vi "Data Read old.vi"(8 "error in (no error)":errorcluster, 10 "Bytes To Read (256)":i32=256, 11 "VISA Refnum in":refnum<visa-resource-name>) -> (0 "error out":errorcluster, 2 "Response Cluster":T1 {"Command ID" format="%x"}, 3 "VISA Refnum out":refnum<visa-resource-name>, 5 "Response String (debug)":string)   [LabVIEW 2020, in "Omega Platinum Series.lvlib"]
uses:
  Omega Platinum Series.lvlib
  Type Defs/Response.ctl
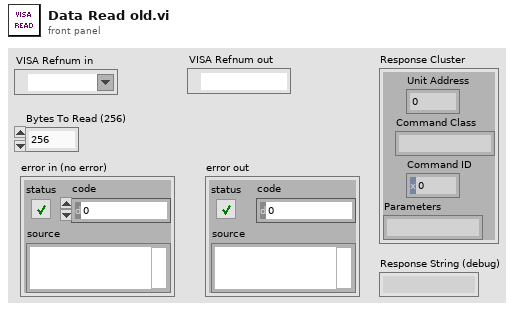
[diagram p1: front panel]
types:
  T1 = typedef "Omega Platinum Series.lvlib/Response.ctl" = cluster{"Unit Address":i32, "Command Class":string, "Command ID":u32, "Parameters":string}
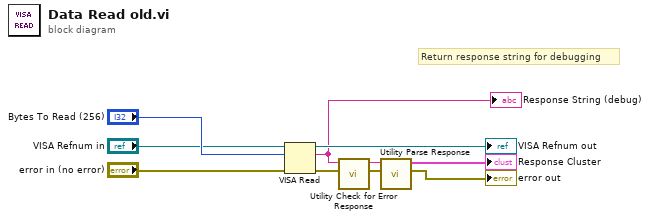
[diagram p0: block diagram]
diagram:
  # "Return response string for debugging"
  n1 = VISA Read(VISA resource name="VISA Refnum in", byte count="Bytes To Read (256)", error in (no error)="error in (no error)") -> (VISA resource name out=→"VISA Refnum out":refnum<visa-resource-name>, read buffer=w7:string, error out=w2:errorcluster)  [unwired: 1 out]
  "Response String (debug)" <- w7
  n2 = call "Utility Check for Error Response.vi"("error in (no error)"=w2, "Response String (in)"=w7) -> ("error out"=w1:errorcluster, "Response String (out)"=w3:string)  [unwired: 8 in]
  n3 = call "Utility Parse Response.vi"("error in (no error)"=w1, "Response String"=w3) -> ("error out"=→"error out":errorcluster, "Response Cluster"=→"Response Cluster":T1)  [unwired: 8 in]
